vi "Manipulation1.vi"() -> ()   [LabVIEW 2017]
panel:
  in  "stop":bool
  in  "Combo Box":string(combo)
  out "Gauge 2":dbl(knob) scale=0.0..10.0
  in  "Y":dbl(slide) scale=0.0..10.0
  in  "X":dbl(slide) scale=0.0..10.0
  in  "calcule":bool
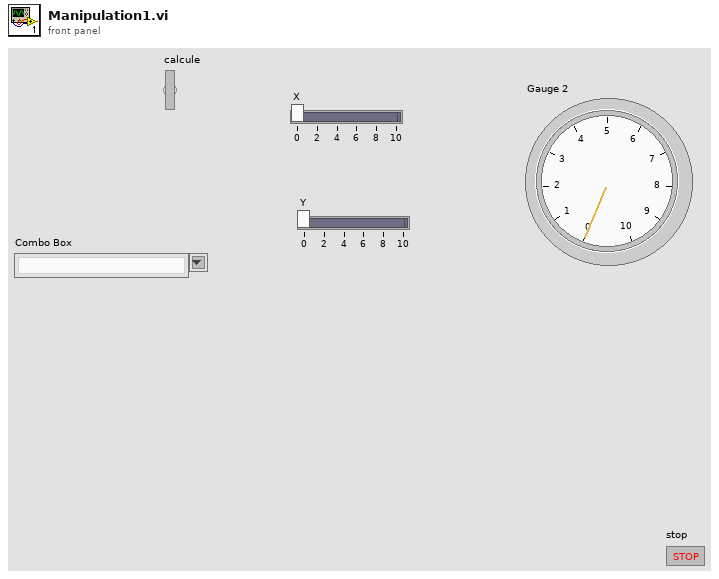
[diagram p1: front panel]
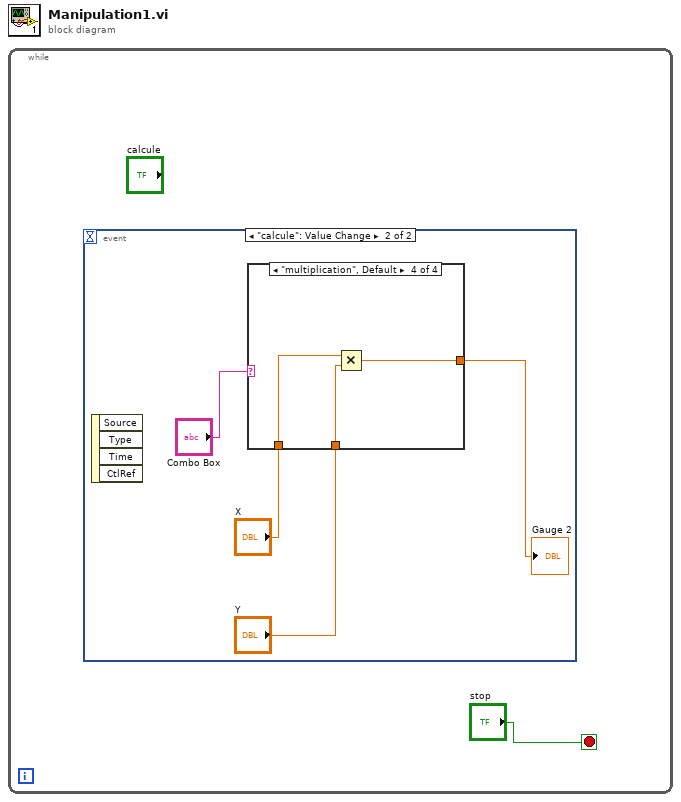
[diagram p0: block diagram]
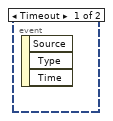
[diagram p2: hidden frame]
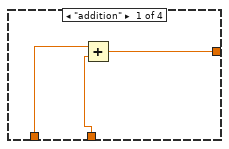
[diagram p3: hidden frame]
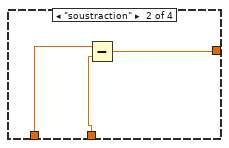
[diagram p4: hidden frame]
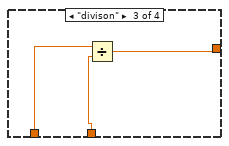
[diagram p5: hidden frame]
diagram:
  n1 = while {
    stop <- "stop" stop-if-true
    n2 = event shown="[1] \"calcule\": Value Change" {
      selector: _ -> [_ _]
      dyn-events: _ -> [_ _]
      timeout: _ -> [_ _]
      event Timeout {
        n3 = event-data() -> ()  [unwired: 1 in, 3 out]
      }
      event "calcule": Value Change {
        n4 = event-data() -> ()  [unwired: 1 in, 4 out]
        n5 = case shown="\"multiplication\", Default" "Combo Box" {
          tunnel: "X" -> [w6 w10 w14 w17]
          tunnel: "Y" -> [w7 w11 w13 w16]
          tunnel: [w8 w9 w12 w15] -> w5
          frame "addition" {
            n6 = Add(x=w6, y=w7) -> (x+y=w8:dbl)
          }
          frame "soustraction" {
            n7 = Subtract(x=w10, y=w11) -> (x-y=w9:dbl)
          }
          frame "divison" {
            n8 = Divide(x=w14, y=w13) -> (x/y=w12:dbl)
          }
          frame "multiplication", Default {
            n9 = Multiply(x=w17, y=w16) -> (x*y=w15:dbl)
          }
        }
        "Gauge 2" <- w5
      }
    }
  }
